vi "FGV_ref.vi"(3 "ref_1D_in":dbl[](array[numeric]), 4 "ref_in":dbl format="%#_13g", 5 "Get (F)":bool) -> (0 "ref_1D_out":dbl[](array[numeric]), 1 "ref_out":dbl)   [LabVIEW 2014]
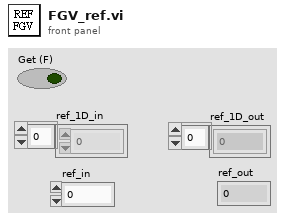
[diagram p1: front panel]
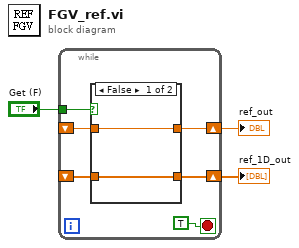
[diagram p0: block diagram]
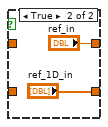
[diagram p2: hidden frame]
diagram:
  n1 = while {
    tunnel: "Get (F)" -> [w8]
    shift-right: [w7] -> w2
    shift-left: _ -> [w6]
    shift-right: [w5] -> w1
    shift-left: _ -> [w4]
    stop <- TRUE stop-if-true
    n2 = case shown="False" w8 {
      tunnel: [w11 "ref_1D_in"] -> w7
      tunnel: w6 -> [w11 _]
      tunnel: [w10 "ref_in"] -> w5
      tunnel: w4 -> [w10 _]
      frame False {
      }
      frame True {
      }
    }
  }
  "ref_1D_out" <- w2
  "ref_out" <- w1
